vi "Apply Friction.vi"(11 "Movable in":refnum<class "Movable.lvclass">) -> (2 "Velocity out":T1, 3 "Movable out":refnum<class "Movable.lvclass">)   [LabVIEW 2021, in "Movable.lvclass"]
doc: "MIT Licence\nCopyright (c) 2024 David Grollier"
uses:
  Movable.lvclass
  Type Def/Velocity.ctl
  Movable.lvclass/Movable.ctl
panel:
  out "s? t:f":T1
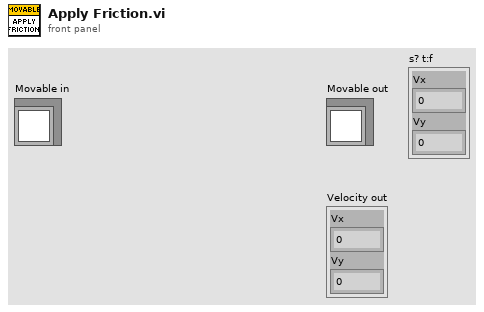
[diagram p1: front panel]
types:
  T1 = typedef "Velocity.ctl" = cluster{"Vx":dbl, "Vy":dbl}
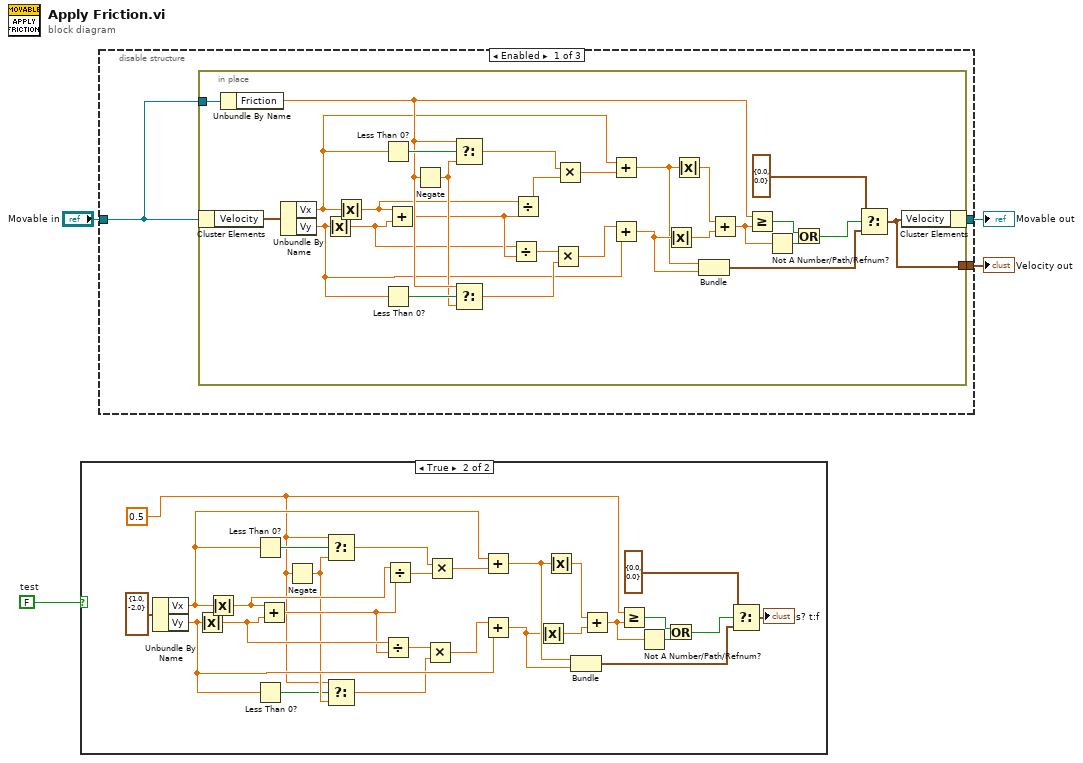
[diagram p0: block diagram]
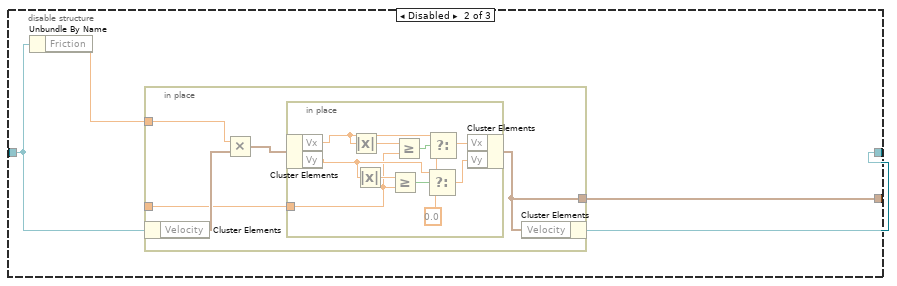
[diagram p3: hidden frame]
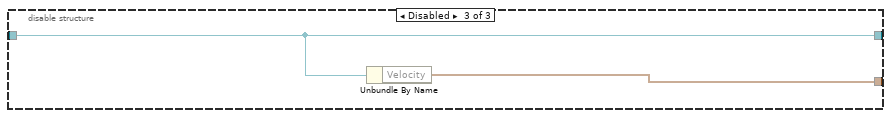
[diagram p4: hidden frame]
diagram:
  w1 = FALSE  # test
  n1 = case shown="True" w1 {
    frame False {
    }
    frame True {
      w6 = 0.5 ("x")
      n2 = Unbundle By Name(T1 {"Vx"=1.0, "Vy"=-2.0} ("input cluster")) -> ("Vx"=w29:dbl, "Vy"=w28:dbl)
      n3 = Absolute Value(x=w28) -> (abs(x)=w27:dbl)
      n4 = Absolute Value(x=w29) -> (abs(x)=w26:dbl)
      n5 = Less Than 0?(x=w29) -> (x < 0?=w9:bool)
      n6 = Less Than 0?(x=w28) -> (x < 0?=w10:bool)
      n7 = Add(x=w26, y=w27) -> (x+y=w12:dbl)
      n8 = Negate(x=w6) -> (-x=w11:dbl)
      n9 = Select(t=w6, s=w9, f=w11) -> (s? t:f=w14:dbl)
      n10 = Select(t=w6, s=w10, f=w11) -> (s? t:f=w18:dbl)
      n11 = Divide(x=w27, y=w12) -> (x/y=w16:dbl)
      n12 = Divide(x=w26, y=w12) -> (x/y=w13:dbl)
      n13 = Multiply(x=w16, y=w18) -> (x*y=w17:dbl)
      n14 = Multiply(x=w14, y=w13) -> (x*y=w15:dbl)
      n15 = Add(x=w29, y=w15) -> (x+y=w20:dbl)
      n16 = Add(x=w17, y=w28) -> (x+y=w19:dbl)
      n17 = Absolute Value(x=w19) -> (abs(x)=w31:dbl)
      n18 = Absolute Value(x=w20) -> (abs(x)=w30:dbl)
      n19 = Bundle(w20, w19) -> (w21:cluster{dbl, dbl})  [unwired: 1 in]
      n20 = Add(x=w30, y=w31) -> (x+y=w22:dbl)
      n21 = Greater Or Equal?(x=w6, y=w22) -> (x >= y?=w24:bool)
      n22 = Not A Number/Path/Refnum?(number/path/refnum=w22) -> (NaN/Path/Refnum?=w23:bool)
      n23 = Or(x=w24, y=w23) -> (x .or. y?=w25:bool)
      n24 = Select(t=T1 {"Vx"=0.0, "Vy"=0.0}, s=w25, f=w21) -> (s? t:f=→"s? t:f":T1)
    }
  }
  n25 = disable-structure shown="Enabled" {
    disable-tunnel: "Movable in" -> [w32 w67 w84]
    disable-tunnel: [w34 w64 w84] -> w3
    disable-tunnel: [w33 w63 w83] -> w2
    frame Enabled {
      n26 = in-place {
        in-place-border: [w59] -> w33
        in-place-border: w32 -> [w62]
        n27 = in-place-cluster #1(w32) -> ("Velocity"=w61:T1)
        n28 = Unbundle By Name(w62) -> ("Friction"=w56:dbl)
        n29 = Unbundle By Name(w61) -> ("Vx"=w37:dbl, "Vy"=w38:dbl)
        n30 = Absolute Value(x=w38) -> (abs(x)=w39:dbl)
        n31 = Absolute Value(x=w37) -> (abs(x)=w40:dbl)
        n32 = Less Than 0?(x=w37) -> (x < 0?=w58:bool)
        n33 = Less Than 0?(x=w38) -> (x < 0?=w57:bool)
        n34 = Add(x=w40, y=w39) -> (x+y=w54:dbl)
        n35 = Negate(x=w56) -> (-x=w55:dbl)
        n36 = Select(t=w56, s=w58, f=w55) -> (s? t:f=w52:dbl)
        n37 = Select(t=w56, s=w57, f=w55) -> (s? t:f=w48:dbl)
        n38 = Divide(x=w39, y=w54) -> (x/y=w50:dbl)
        n39 = Divide(x=w40, y=w54) -> (x/y=w53:dbl)
        n40 = Multiply(x=w50, y=w48) -> (x*y=w49:dbl)
        n41 = Multiply(x=w52, y=w53) -> (x*y=w51:dbl)
        n42 = Add(x=w37, y=w51) -> (x+y=w46:dbl)
        n43 = Add(x=w49, y=w38) -> (x+y=w47:dbl)
        n44 = Absolute Value(x=w47) -> (abs(x)=w35:dbl)
        n45 = Absolute Value(x=w46) -> (abs(x)=w36:dbl)
        n46 = Bundle(w46, w47) -> (w45:cluster{dbl, dbl})  [unwired: 1 in]
        n47 = Add(x=w36, y=w35) -> (x+y=w44:dbl)
        n48 = Greater Or Equal?(x=w56, y=w44) -> (x >= y?=w42:bool)
        n49 = Not A Number/Path/Refnum?(number/path/refnum=w44) -> (NaN/Path/Refnum?=w43:bool)
        n50 = Or(x=w42, y=w43) -> (x .or. y?=w41:bool)
        n51 = Select(t=T1 {"Vx"=0.0, "Vy"=0.0}, s=w41, f=w45) -> (s? t:f=w59:T1)
        n52 = in-place-cluster #1("Velocity"=w59) -> (w34:refnum<class "Movable.lvclass">)
      }
    }
    frame Disabled {
      n53 = Unbundle By Name(w67) -> ("Friction"=w66:dbl)
      n54 = in-place {
        in-place-border: w66 -> [w70]
        in-place-border: [w69] -> w65
        in-place-border: [w68] -> w63
        n55 = in-place-cluster #2(w67) -> ("Velocity"=w72:T1)
        n56 = Multiply(x=w70, y=w72) -> (x*y=w71:T1)
        n57 = in-place {
          in-place-border: w69 -> [w75]
          w80 = 0.0 ("f")
          n58 = in-place-cluster #3(w71) -> ("Vx"=w77:dbl, "Vy"=w76:dbl)
          n59 = Absolute Value(x=w77) -> (abs(x)=w81:dbl)
          n60 = Absolute Value(x=w76) -> (abs(x)=w82:dbl)
          n61 = Greater Or Equal?(x=w82, y=w75) -> (x >= y?=w78:bool)
          n62 = Greater Or Equal?(x=w81, y=w75) -> (x >= y?=w79:bool)
          n63 = Select(t=w76, s=w78, f=w80) -> (s? t:f=w74:dbl)
          n64 = Select(t=w77, s=w79, f=w80) -> (s? t:f=w73:dbl)
          n65 = in-place-cluster #3("Vx"=w73, "Vy"=w74) -> (w68:T1)
        }
        n66 = in-place-cluster #2("Velocity"=w68) -> (w64:refnum<class "Movable.lvclass">)
      }
    }
    frame Disabled {
      n67 = Unbundle By Name(w84) -> ("Velocity"=w83:T1)
    }
  }
  "Movable out" <- w3
  "Velocity out" <- w2
